vi "main timed loop.vi"(10 "cmd fifo":refnum<k33>, 11 "Engine Data Out in":T2={"timed loop timer source"={"Processor"=0, "Priority"=0, "timing source dt"=0, "timer source"=refnum}, "control loop data"={"engine tag bus"={"Double"=[], "Single"=[], "I64"=[], "I32"=[], "I16"=[], "I8"=[], "U64"=[], "U32"=[], "U16"=[], "U8"=[], "Boolean"=[], "String"=[], "Array of Double"=[], "Array of Single"=[], "Array of I64"=[], "Array of I32"=[], "Array of I16"=[], "Array of I8"=[], "Array of U64"=[], "Array of U32"=[], "Array of U16"=[], "Array of U8"=[], "Array of Boolean"=[], "Array of String"=[]}, "engine schedule"={"module run flags"=[], "decimation schedule"={"decimations"=[], "offsets"=[]}}, "module information"=[]}, "status reporting"={"late? index (bool)"=-1, "late count index (U32)"=-1, "dt (ns) index (U64)"=-1}} {"control loop data"."module information"."GUID"."Lo" format="%.0x"; "control loop data"."module information"."GUID"."Hi" format="%.0x"}) -> (0 "error out":errorcluster, 2 "desired state":T1, 3 "Engine Data Out out":T2={"timed loop timer source"={"Processor"=0, "Priority"=0, "timing source dt"=0, "timer source"=refnum}, "control loop data"={"engine tag bus"={"Double"=[], "Single"=[], "I64"=[], "I32"=[], "I16"=[], "I8"=[], "U64"=[], "U32"=[], "U16"=[], "U8"=[], "Boolean"=[], "String"=[], "Array of Double"=[], "Array of Single"=[], "Array of I64"=[], "Array of I32"=[], "Array of I16"=[], "Array of I8"=[], "Array of U64"=[], "Array of U32"=[], "Array of U16"=[], "Array of U8"=[], "Array of Boolean"=[], "Array of String"=[]}, "engine schedule"={"module run flags"=[], "decimation schedule"={"decimations"=[], "offsets"=[]}}, "module information"=[]}, "status reporting"={"late? index (bool)"=-1, "late count index (U32)"=-1, "dt (ns) index (U64)"=-1}} {"control loop data"."module information"."GUID"."Lo" format="%.0x"; "control loop data"."module information"."GUID"."Hi" format="%.0x"})   [LabVIEW 2013, in "Standard Engine Runtime.lvclass"]
uses:
  Standard Engine Runtime.lvclass
  Commands.ctl
  <vilib>/Platform/TimedLoop/XDataNode/wakeup.ctl
  <vilib>/Platform/TimedLoop/XDataNode/XDNodeRunTimeDep.lvlib
  <vilib>/Platform/TimedLoop/XDataNode/nitl_modes.ctl
  <vilib>/Platform/TimedLoop/XDataNode/timing_clust.ctl
  <vilib>/platform/TimedLoop/XDataNode/XDataNode.xnode
  async executor/async executor.lvlib
  <vilib>/NI/Module Timing Source/timing source/TBM timing source.lvclass
  <vilib>/NI/Tag Bus/table/data table.ctl
  <vilib>/NI/Tag Bus/table/data table.lvlib
  <vilib>/NI/Tag Bus Module Framework/runtime/TBM module execution interface.lvclass
  <vilib>/NI/Tag Bus/tag/Data Type.ctl
  <vilib>/NI/Tag Bus/tag/tag descriptor.lvclass
  <vilib>/NI/Tag Bus/table/transfer specification.ctl
  Configuration/Error Actions.ctl
  Configuration/Standard Engine Configuration.lvclass
  Engine Data.ctl
  engine state.ctl
  timed loop timing sources.ctl
  <vilib>/NI/Tag Bus/buffer exchange/buffer reference.ctl
  <vilib>/NI/Tag Bus/buffer exchange/tag bus buffer exchange.lvlib
  <vilib>/NI/Tag Bus/buffer exchange/buffer exchange.ctl
  async executor/asynchronous executor reference.ctl
  module run state.ctl
  module method data.ctl
  fault handling spec.ctl
  <vilib>/NI/Configuration Framework/serializable configuration/Numeric GUID.ctl
  <vilib>/NI/Configuration Framework/serializable configuration/NISE_CEF_serializable configuration.lvclass
  <vilib>/NI/Tag Bus Module Framework/module configuration/TBM module configuration.lvclass
  full module data.ctl
  engine decimation schedule.ctl
  engine run schedule.ctl
  control loop data.ctl
  status reporting data.ctl
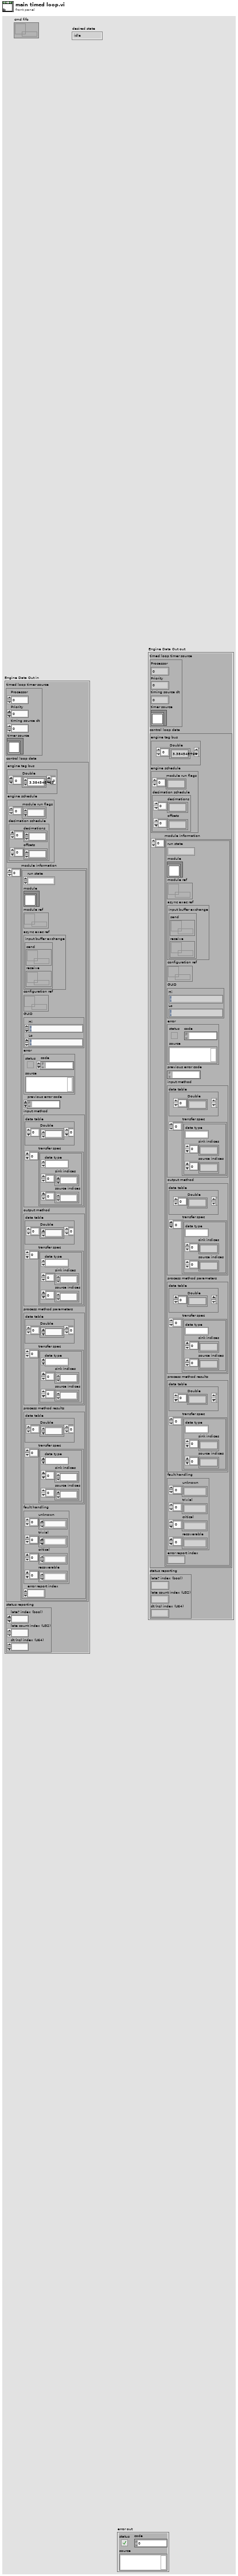
[diagram p1: front panel]
types:
  T1 = typedef "Standard Engine Runtime.lvclass/engine state.ctl" = enum16{"idle", "configured", "running", "safe state", "exit"}
  T2 = typedef "Standard Engine Runtime.lvclass/Engine Data.ctl" = cluster{"timed loop timer source":T3, "control loop data":T4, "status reporting":T18}
  T3 = typedef "Standard Engine Runtime.lvclass/timed loop timing sources.ctl" = cluster{"Processor":i32, "Priority":i32, "timing source dt":u32, "timer source":refnum<class "TBM timing source.lvclass">}
  T4 = typedef "Standard Engine Runtime.lvclass/control loop data.ctl" = cluster{"engine tag bus":T5, "engine schedule":T6, "module information":T8[]}
  T5 = typedef "tag bus.lvlib/data table.lvlib/data table.ctl" = cluster{"Double":dbl[], "Single":sgl[], "I64":i64[], "I32":i32[], "I16":i16[], "I8":i8[], "U64":u64[], "U32":u32[], "U16":u16[], "U8":u8[], "Boolean":bool[], "String":string[], "Array of Double":cluster{"DBL Array":dbl[]}[], "Array of Single":cluster{"SGL Array":sgl[]}[], "Array of I64":cluster{"I64 Array":i64[]}[], "Array of I32":cluster{"I32 Array":i32[]}[], "Array of I16":cluster{"I16 Array":i16[]}[], "Array of I8":cluster{"I8 Array":i8[]}[], "Array of U64":cluster{"U64 Array":u64[]}[], "Array of U32":cluster{"U32 Array":u32[]}[], "Array of U16":cluster{"U16 Array":u16[]}[], "Array of U8":cluster{"U8 Array":u8[]}[], "Array of Boolean":cluster{"Boolean Array":bool[]}[], "Array of String":cluster{"String Array":string[]}[]}
  T6 = typedef "Standard Engine Runtime.lvclass/engine run schedule.ctl" = cluster{"module run flags":u8[], "decimation schedule":T7}
  T7 = typedef "Standard Engine Runtime.lvclass/engine decimation schedule.ctl" = cluster{"decimations":u16[], "offsets":u16[]}
  T8 = typedef "Standard Engine Runtime.lvclass/full module data.ctl" = cluster{"run state":T9, "module":refnum<class "TBM module execution interface.lvclass">, "module ref":refnum<data-value>, "async exec ref":T10, "configuration ref":refnum<data-value>, "GUID":T12, "error":errorcluster, "previous error code":i32, "input method":T13, "output method":T13, "process method parameters":T13, "process method results":T13, "fault handling":T16, "error report index ":i32}
  T9 = typedef "Standard Engine Runtime.lvclass/module run state.ctl" = enum16{"sync", "async"}
  T10 = typedef "async executor.lvlib/asynchronous executor reference.ctl" = cluster{"input buffer exchange":T11}
  T11 = typedef "tag bus buffer exchange.lvlib/buffer exchange.ctl" = cluster{"send":refnum<k33>, "receive":refnum<k33>}
  T12 = typedef "NISE_CEF_serializable configuration.lvclass/Numeric GUID.ctl" = cluster{"Hi":u64, "Lo":u64}
  T13 = typedef "Standard Engine Runtime.lvclass/module method data.ctl" = cluster{"data table":T5, "transfer spec":T14[]}
  T14 = typedef "tag bus.lvlib/data table.lvlib/transfer specification.ctl" = cluster{"data type":T15, "sink indices":i32[], "source indices":i32[]}
  T15 = typedef "tag bus.lvlib/tag descriptor.lvclass/Data Type.ctl" = enum16{"Double", "Single", "I64", "I32", "I16", "I8", "U64", "U32", "U16", "U8", "Boolean", "String", "Array of Double", "Array of Single", "Array of I64", "Array of I32", "Array of I16", "Array of I8", "Array of U64", "Array of U32", "Array of U16", "Array of U8", "Array of Boolean", "Array of String"}
  T16 = typedef "Standard Engine Runtime.lvclass/fault handling spec.ctl" = cluster{"unknown":T17[], "trivial":T17[], "critical":T17[], "recoverable":T17[]}
  T17 = typedef "Standard Engine Configuration.lvclass/Error Actions.ctl" = enum16{"Clear", "Notify", "Stop Component", "Stop Engine", "Safe State", "Attempt Recovery"}
  T18 = typedef "Standard Engine Runtime.lvclass/status reporting data.ctl" = cluster{"late? index (bool)":i32, "late count index (U32)":i32, "dt (ns) index (U64)":i32}
  T19 = typedef "Standard Engine Runtime.lvclass/Module Execution Info.ctl" = cluster{"Tag Bus Modules":refnum<class "TBM module execution interface.lvclass">[], "Execute?":bool[], "Input Method Indices":i32[], "Process Method Indices":i32[], "Output Method Indices":i32[], "Input Transfer Specifications":T20[], "Parameter Transfer Specifications":T20[], "Result Transfer Specifications":T20[], "Output Transfer Specifications":T20[], "Module Errors":errorcluster[], "Module Decimation":T21[], "Module Decimation Indices":i32[], "Error Queue":refnum<queue>, "Module Error Configuration":T22[], "Module Errors (n-1)":errorcluster[], "error responses":T25}
  T20 = typedef "Standard Engine Runtime.lvclass/Data Table with Transfer Spec.ctl" = cluster{"Data Table":T5, "Transfer Specification":T14[]}
  T21 = typedef "Standard Engine Configuration.lvclass/Module Decimation.ctl" = cluster{"Decimation":u16, "Offset":u16, "sort order":i32, "async?":bool}
  T22 = typedef "Standard Engine Configuration.lvclass/Module Error Configuration.ctl" = cluster{"Module Error Configuration":T23[]}
  T23 = typedef "Standard Engine Configuration.lvclass/Error Actions By Category.ctl" = cluster{"error classification":T24, "Error Actions":T17[]}
  T24 = typedef "TBM module execution interface.lvclass/error classification.ctl" = enum16{"unknown", "none", "trivial", "recoverable", "critical"}
  T25 = typedef "Standard Engine Configuration.lvclass/error responses.ctl" = cluster{"unknown":T26, "trivial":T26, "critical":T26, "recoverable":T26}
  T26 = typedef "Standard Engine Configuration.lvclass/error options.ctl" = cluster{"clear":bool, "notify":bool, "remove module":bool, "abort engine":bool, "go to safe state":bool, "recover module":bool}
  T27 = typedef "Standard Engine Runtime.lvclass/async execution info.ctl" = cluster{"Tag Bus Modules":T28[], "Execute?":bool[], "Input Method Indices":i32[], "Process Method Indices":i32[], "Output Method Indices":i32[], "Input Transfer Specifications":T20[], "Parameter Transfer Specifications":T20[], "Result Transfer Specifications":T20[], "Output Transfer Specifications":T20[], "Module Errors":errorcluster[], "Module Decimation":T21[], "Module Decimation Indices":i32[], "Error Queue":refnum<queue>, "Module Error Configuration":T22[], "comm errors":errorcluster[]}
  T28 = typedef "Standard Engine Runtime.lvclass/asynchronous process data.ctl" = cluster{"thread reference":refnum<vi>, "cmd notification":refnum<k33>, "execution period (ms)":i32, "input from component":refnum<queue>, "input to component":refnum<queue>, "output from component":refnum<queue>, "output to component":refnum<queue>, "process input from component":refnum<queue>, "process input to component":refnum<queue>, "process result from component":refnum<queue>, "process result to component":refnum<queue>, "execution settings":T29, "error fifo":refnum<k33>}
  T29 = typedef "TBM module execution interface.lvclass/execution settings.ctl" = cluster{"reads inputs":bool, "processes data":bool, "writes outputs":bool}
  T30 = typedef "XDNodeRunTimeDep.lvlib/timing_clust.ctl" = cluster{"Expected End [f-1]":u64, "Actual End [f-1]":u64, "Finished Late? [f-1]":bool, "Expected End [i-1]":u64, "Actual End [i-1]":u64, "Finished Late? [i-1]":bool, "Expected Start [i]":u64, "Actual Start [i]":u64, "Expected Start [f]":u64, "Actual Start [f]":u64, "Source Name":string, "Structure Name":string, "Period":i64, "Deadline":i64, "Offset":i64, "Start":i64, "Priority":i32, "Timeout":i32, "Mode":T31, "Wakeup Reason":T32, "Error":errorcluster, "Source Type":string, "Secondary Source Type":string, "Global End Time":u64, "Global Start Time":u64, "Frame Duration":u64, "Iteration Duration":u64, "Assigned CPU":i32, "I/O Scan Engine Mode":u32}
  T31 = typedef "XDNodeRunTimeDep.lvlib/nitl_modes.ctl" = enum32{"No Change", "Process missed periods, maintain original phase", "Discard missed periods, maintain original phase", "Process missed periods, ignore original phase", "Discard missed periods, ignore original phase"}
  T32 = typedef "XDNodeRunTimeDep.lvlib/wakeup.ctl" = enum32{"Normal", "Aborted", "Asynchronous wakeup", "Timing source error", "Timed loop error", "Timeout"}
  T33 = typedef "Commands.ctl" = enum16{"Initialize", "Start", "Pause", "Safe State", "Normal", "Stop", "Shutdown"}
  T34 = typedef "Module Execution Info.ctl" = cluster{"Tag Bus Modules":refnum<class "TBM module execution interface.lvclass">[], "Execute?":bool[], "Input Method Indices":i32[], "Process Method Indices":i32[], "Output Method Indices":i32[], "Input Transfer Specifications":T35[], "Parameter Transfer Specifications":T35[], "Result Transfer Specifications":T35[], "Output Transfer Specifications":T35[], "Module Errors":errorcluster[], "Module Decimation":T21[], "Module Decimation Indices":i32[], "Error Queue":refnum<queue>, "Module Error Configuration":T22[], "Module Errors (n-1)":errorcluster[], "error responses":T25}
  T35 = typedef "Data Table with Transfer Spec.ctl" = cluster{"Data Table":T5, "Transfer Specification":T14[]}
  T36 = typedef "async executor.lvlib/async execution info.ctl" = cluster{"Tag Bus Modules":T37[], "Execute?":bool[], "Input Method Indices":i32[], "Process Method Indices":i32[], "Output Method Indices":i32[], "Input Transfer Specifications":T35[], "Parameter Transfer Specifications":T35[], "Result Transfer Specifications":T35[], "Output Transfer Specifications":T35[], "Module Errors":errorcluster[], "Module Decimation":T21[], "Module Decimation Indices":i32[], "Error Queue":refnum<queue>, "Module Error Configuration":T22[], "comm errors":errorcluster[]}
  T37 = typedef "async executor.lvlib/asynchronous process data.ctl" = cluster{"thread reference":refnum<vi>, "cmd notification":refnum<k33>, "execution period (ms)":i32, "input from component":refnum<queue>, "input to component":refnum<queue>, "output from component":refnum<queue>, "output to component":refnum<queue>, "process input from component":refnum<queue>, "process input to component":refnum<queue>, "process result from component":refnum<queue>, "process result to component":refnum<queue>, "execution settings":T29, "error fifo":refnum<k33>}
  T38 = typedef "worker pool.lvlib/worker comms.ctl" = cluster{"command fifo":refnum<k33>, "request fifos":T39, "response fifos":T40}
  T39 = typedef "worker pool.lvlib/request fifos.ctl" = cluster{"recovery":refnum<k33>}
  T40 = typedef "worker pool.lvlib/response fifos.ctl" = cluster{"recovery":refnum<k33>}
  T41 = typedef "Standard Engine Runtime.lvclass/Commands.ctl" = enum16{"Initialize", "Start", "Pause", "Safe State", "Normal", "Stop", "Shutdown"}
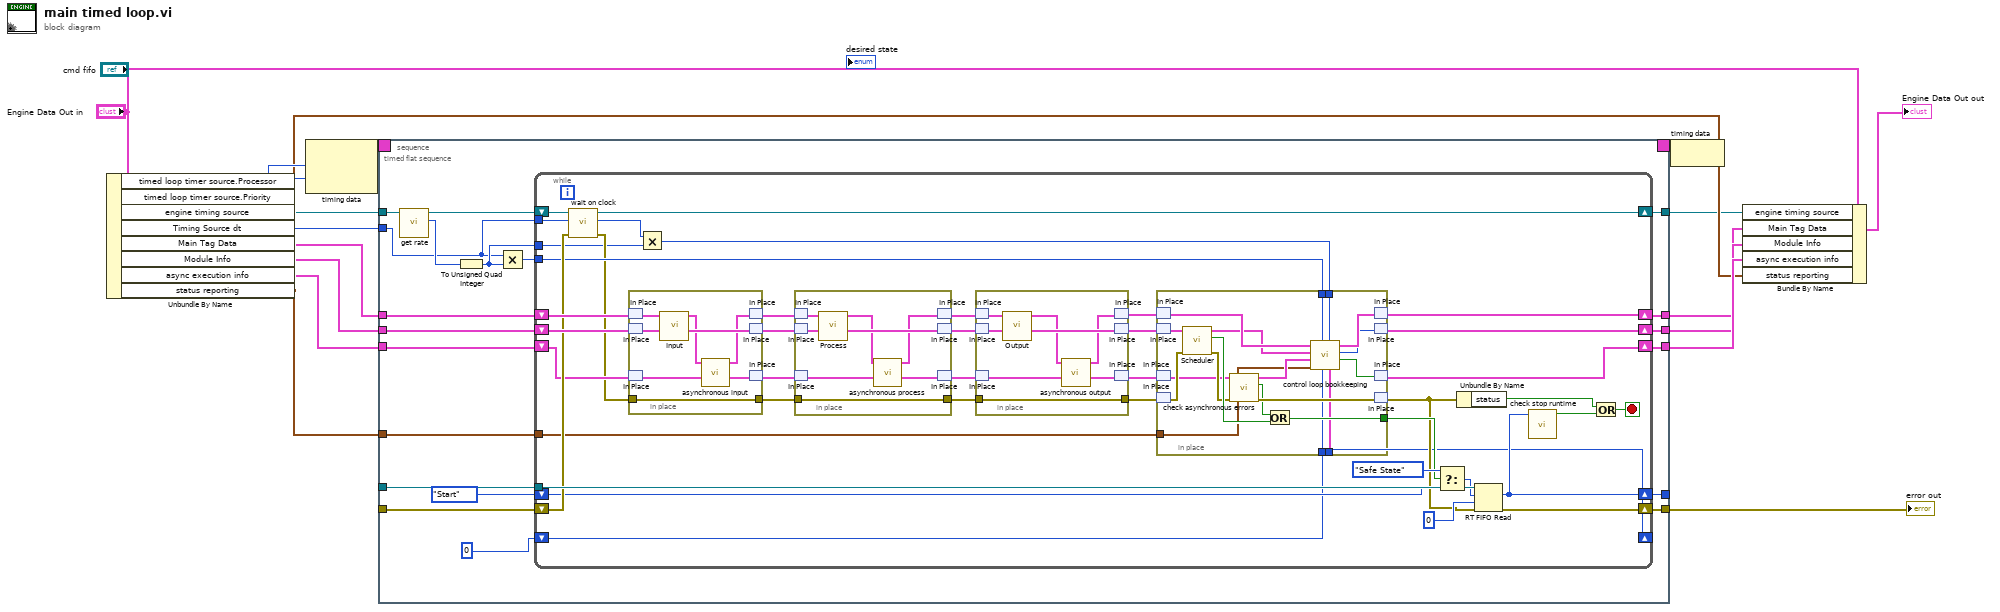
[diagram p0: block diagram]
diagram:
  n1 = Unbundle By Name("Engine Data Out in") -> ("timed loop timer source.Processor"=w15:i32, "timed loop timer source.Priority"=w16:i32, "engine timing source"=w5:refnum<class "TBM timing source.lvclass">, "Timing Source dt"=w17:u32, "Main Tag Data"=w6:T5, "Module Info"=w7:T19, "async execution info"=w8:T27, "status reporting"=w10:T18)
  n2 = node-c288(w15, w16) -> (w19:T30)
  n3 = timed-sequence {
    timing: w19 -> [_]
    timing-out: [_] -> w18
    tunnel: [w33] -> w1
    tunnel: [w32] -> _
    tunnel: [w31] -> w4
    tunnel: w5 -> [w21]
    tunnel: w6 -> [w30]
    tunnel: w7 -> [w29]
    tunnel: w8 -> [w28]
    tunnel: [w27] -> w9
    tunnel: w10 -> [w26]
    tunnel: [w25] -> w11
    tunnel: [w24] -> w12
    tunnel: [w23] -> w13
    tunnel: [w22] -> w14
    tunnel: w17 -> [w20]
    n4 = timed-flat-sequence {
      tunnel: w33 -> [w53]
      tunnel: [w52] -> w32
      tunnel: [w51] -> w31
      tunnel: w30 -> [w50]
      tunnel: w29 -> [w49]
      tunnel: w28 -> [w48]
      tunnel: [w47] -> w27
      tunnel: w26 -> [w46]
      tunnel: [w45] -> w25
      tunnel: [w44] -> w24
      tunnel: [w43] -> w23
      tunnel: w22 -> [w39]
      tunnel: w21 -> [w38]
      tunnel: w20 -> [w34]
      n5 = call-dynamic "get rate.vi"("timing source in"=w38) -> ("period (ns)"=w36:i64, "timing source out"=w41:refnum<class "TBM timing source.lvclass">)  [unwired: 8 in, 1 out]
      n6 = To Unsigned Quad Integer(1:w36) -> (0:w35:u64)
      n7 = Multiply(x=w34, y=w35) -> (x*y=w37:u64)
      n8 = while {
        tunnel: w53 -> [w85]
        shift-right: [w87] -> w52
        shift-left: Commands."Start" ("Commands") -> [w74]
        shift-right: [w68] -> w45
        shift-left: w50 -> [w94]
        shift-right: [w88] -> w44
        shift-left: w49 -> [w93]
        shift-right: [w84] -> w51
        shift-left: w39 -> [w81]
        shift-right: [w80] -> w47
        shift-left: w41 -> [w82]
        tunnel: w37 -> [w67]
        shift-right: [w75] -> w43
        shift-left: w48 -> [w79]
        tunnel: w46 -> [w66]
        shift-right: [w65] -> _
        shift-left: u32 0 ("late count out") -> [w64]
        tunnel: w35 -> [w59]
        tunnel: w34 -> [w54]
        stop <- w56 stop-if-true
        n9 = call-dynamic "wait on clock.vi"("error in"=w81, "dt"=w54, "timing source in"=w82) -> ("error out"=w63:errorcluster, "ticks since last call"=w58:u32, "timing source out"=w80:refnum<class "TBM timing source.lvclass">)  [unwired: 6 in]
        n10 = in-place {
          in-place-border: w63 -> [w134]
          in-place-border: [w134] -> w60
          n11 = in-place-match #1(w94) -> (w133:T5)
          n12 = in-place-match #2(w93) -> (w138:T19)
          n13 = in-place-match #3(w79) -> (w136:T27)
          n14 = call "Input.vi"("Module Info In"=w138, "Engine Tags In"=w133) -> ("Module Info Out"=w137:T34, "Engine Tags Out"=w132:T5)  [unwired: 8 in]
          n15 = call "asynchronous input.vi"("Module Info In"=w136, "Engine Tags In"=w132) -> ("Module Info Out"=w135:T36, "Engine Tags Out"=w131:T5)  [unwired: 8 in]
          n16 = in-place-match #1(w131) -> (w92:T5)
          n17 = in-place-match #2(w137) -> (w91:T19)
          n18 = in-place-match #3(w135) -> (w78:T27)
        }
        n19 = Multiply(x=w58, y=w59) -> (x*y=w57:u64)
        n20 = in-place {
          in-place-border: [w123] -> w61
          in-place-border: w60 -> [w123]
          n21 = in-place-match #4(w92) -> (w129:T5)
          n22 = in-place-match #5(w91) -> (w130:T19)
          n23 = in-place-match #6(w78) -> (w127:T27)
          n24 = call "Process.vi"("Module Info In"=w130, "Engine Tags In"=w129) -> ("Module Info Out"=w128:T34, "Engine Tags Out"=w126:T5)  [unwired: 8 in]
          n25 = call "asynchronous process.vi"("Module Info In"=w127, "Engine Tags In"=w126) -> ("Module Info Out"=w125:T36, "Engine Tags Out"=w124:T5)  [unwired: 8 in]
          n26 = in-place-match #4(w124) -> (w83:T5)
          n27 = in-place-match #5(w128) -> (w90:T19)
          n28 = in-place-match #6(w125) -> (w77:T27)
        }
        n29 = in-place {
          in-place-border: [w115] -> w62
          in-place-border: w61 -> [w115]
          n30 = in-place-match #7(w83) -> (w122:T5)
          n31 = in-place-match #8(w90) -> (w121:T19)
          n32 = in-place-match #9(w77) -> (w119:T27)
          n33 = call "Output.vi"("Module Info In"=w121, "Engine Tags In"=w122) -> ("Module Info Out"=w120:T34, "Engine Tags Out"=w117:T5)  [unwired: 8 in]
          n34 = call "asynchronous output.vi"("Module Info In"=w119, "Engine Tags In"=w117) -> ("Module Info Out"=w118:T36, "Engine Tags Out"=w116:T5)  [unwired: 8 in]
          n35 = in-place-match #7(w116) -> (w69:T5)
          n36 = in-place-match #8(w120) -> (w89:T19)
          n37 = in-place-match #9(w118) -> (w76:T27)
        }
        n38 = in-place {
          in-place-border: [w110] -> w71
          in-place-border: w67 -> [w97]
          in-place-border: w57 -> [w96]
          in-place-border: w66 -> [w98]
          in-place-border: [w100] -> w65
          in-place-border: w64 -> [w99]
          n39 = in-place-match #10(w69) -> (w106:T5)
          n40 = in-place-match #11(w89) -> (w107:T19)
          n41 = in-place-match #12(w76) -> (w108:T27)
          n42 = in-place-match #13(w62) -> (w114:errorcluster)
          n43 = call "Scheduler.vi"("error in"=w114, "Module Info In"=w107) -> ("error out"=w112:errorcluster, "Safe State?"=w113:bool, "Module Info Out"=w105:T34)  [unwired: 7 in]
          n44 = call "check asynchronous errors.vi"("error in"=w112, "Module Info In"=w108) -> ("error out"=w111:errorcluster, "safe state?"=w109:bool, "Module Info Out"=w102:T36)  [unwired: 7 in]
          n45 = Or(x=w109, y=w113) -> (x .or. y?=w110:bool)
          n46 = call "control loop bookkeeping.vi"("ns since last call"=w96, "fault fifo"=w99, "finished late?"=w97, "engine error in"=w98, "status reporting in"=w102, "late count in"=w105, "control loop data in"=w106) -> ("safe state?"=w101:bool, "late count out"=w103:u32, "control loop data out"=w104:T4, "worker pool reference"=w100:T38)  [unwired: 1 out]
          n47 = in-place-match #10(w104) -> (w68:T5)
          n48 = in-place-match #11(w103) -> (w88:T19)
          n49 = in-place-match #12(w101) -> (w75:T27)
          n50 = in-place-match #13(w111) -> (w70:errorcluster)
        }
        n51 = Select(t=Commands."Safe State" ("y"), s=w71, f=w74) -> (s? t:f=w73:T41)
        n52 = Unbundle By Name(w70) -> ("status"=w55:bool)
        n53 = RT FIFO Read(0:w85, 1:w73, 2:0 ("timeout in ms (0)"), 3:w70) -> (9:w87:T41, 11:w84:errorcluster)  [unwired: 3 out]
        n54 = call "check stop runtime.vi"("Commands"=w87) -> ("stop?"=w86:bool)  [unwired: 10 in]
        n55 = Or(x=w55, y=w86) -> (x .or. y?=w56:bool)
      }
    }
  }
  "error out" <- w4
  n56 = node-c288(w18) -> ()
  n57 = Bundle By Name(cluster="Engine Data Out in", "engine timing source"=w9, "Main Tag Data"=w11, "Module Info"=w12, "async execution info"=w13, "status reporting"=w10) -> (→"Engine Data Out out":T2)
